vi "findDirectPath.vi"(8 "error in (no error)":errorcluster, 10 "goal platform":i32, 11 "start platform":i32) -> (0 "error out":errorcluster, 1 "vector \nlength":dbl, 2 "vector\nangle":dbl, 3 "path":dbl[](array[numeric]))   [LabVIEW 2017]
panel:
  out "empty?":bool
  out "direct path - first index is row\nof paths through start, \nsecond is location of \ngoal in path":i32[][](array[numeric])
  out "start indices":i32[](array[numeric])
  out "goal indices":i32[](array[numeric])
  out "paths through goal":dbl[][](array[numeric])
  out "paths through start":dbl[][](array[numeric])
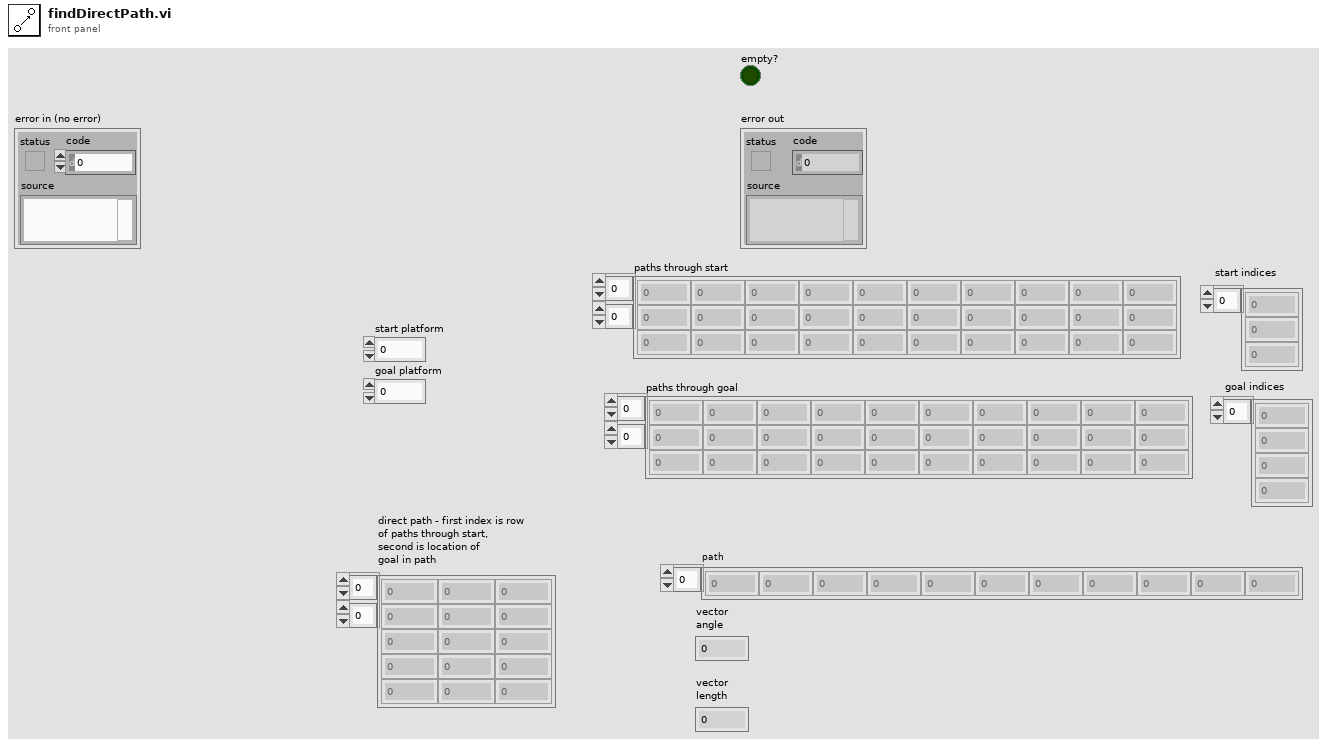
[diagram p1: front panel]
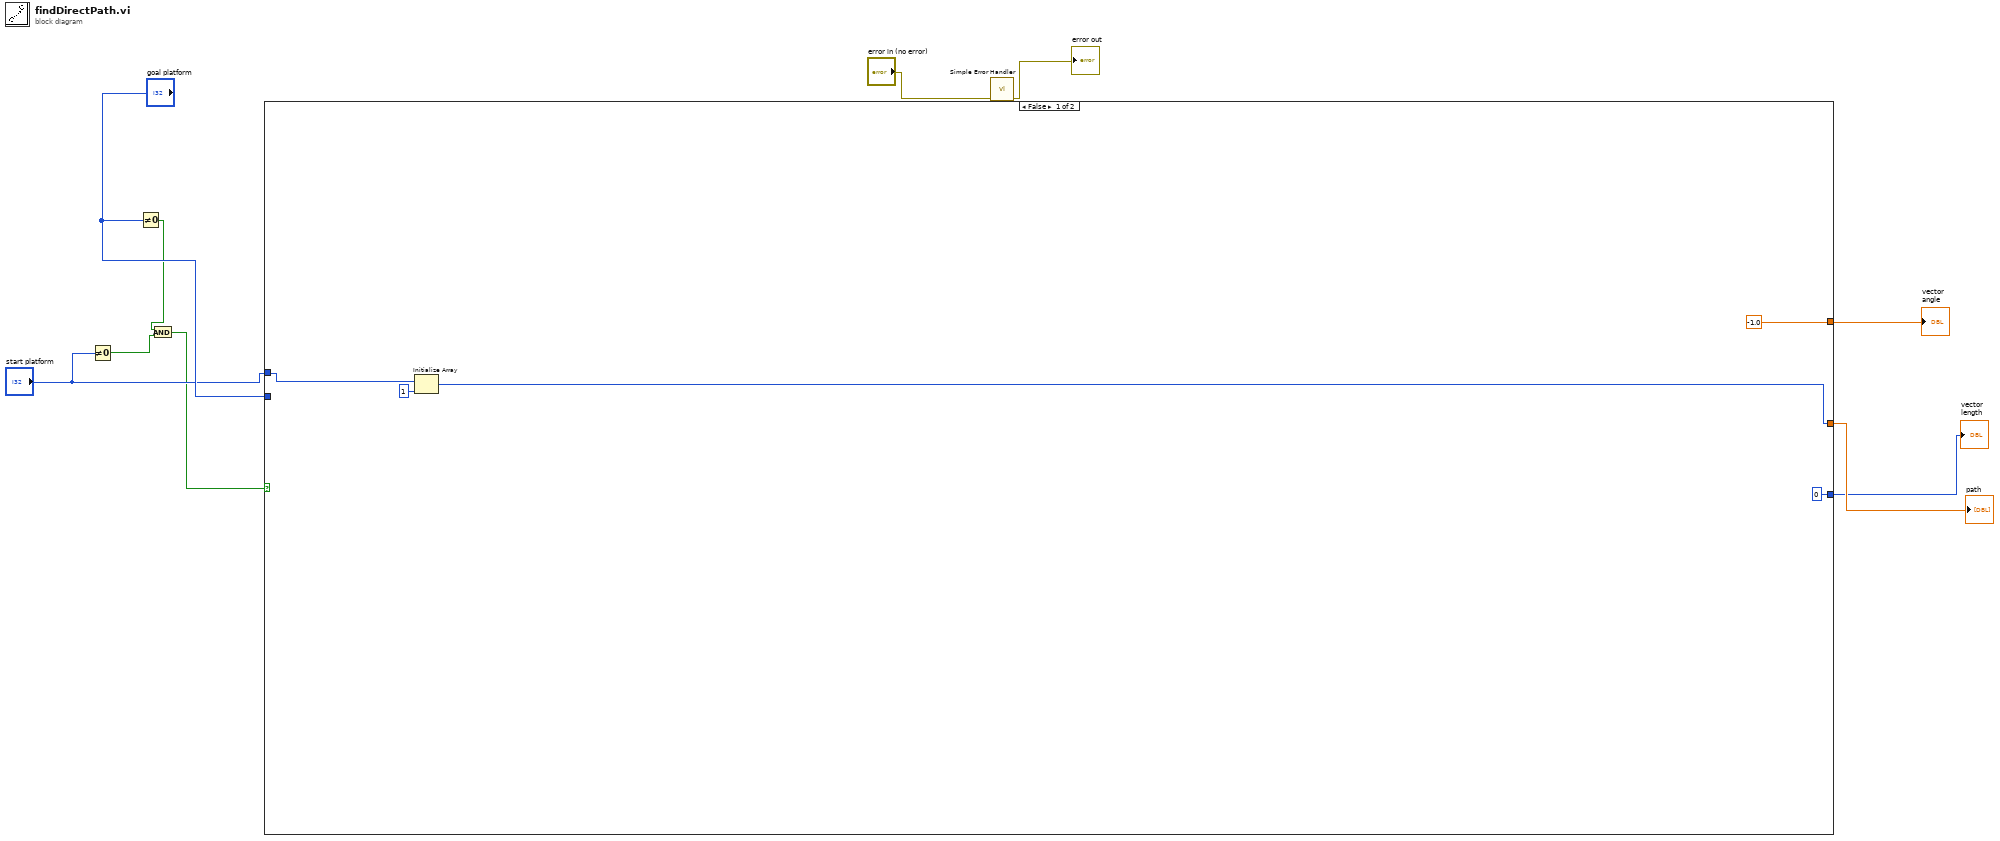
[diagram p0: block diagram]
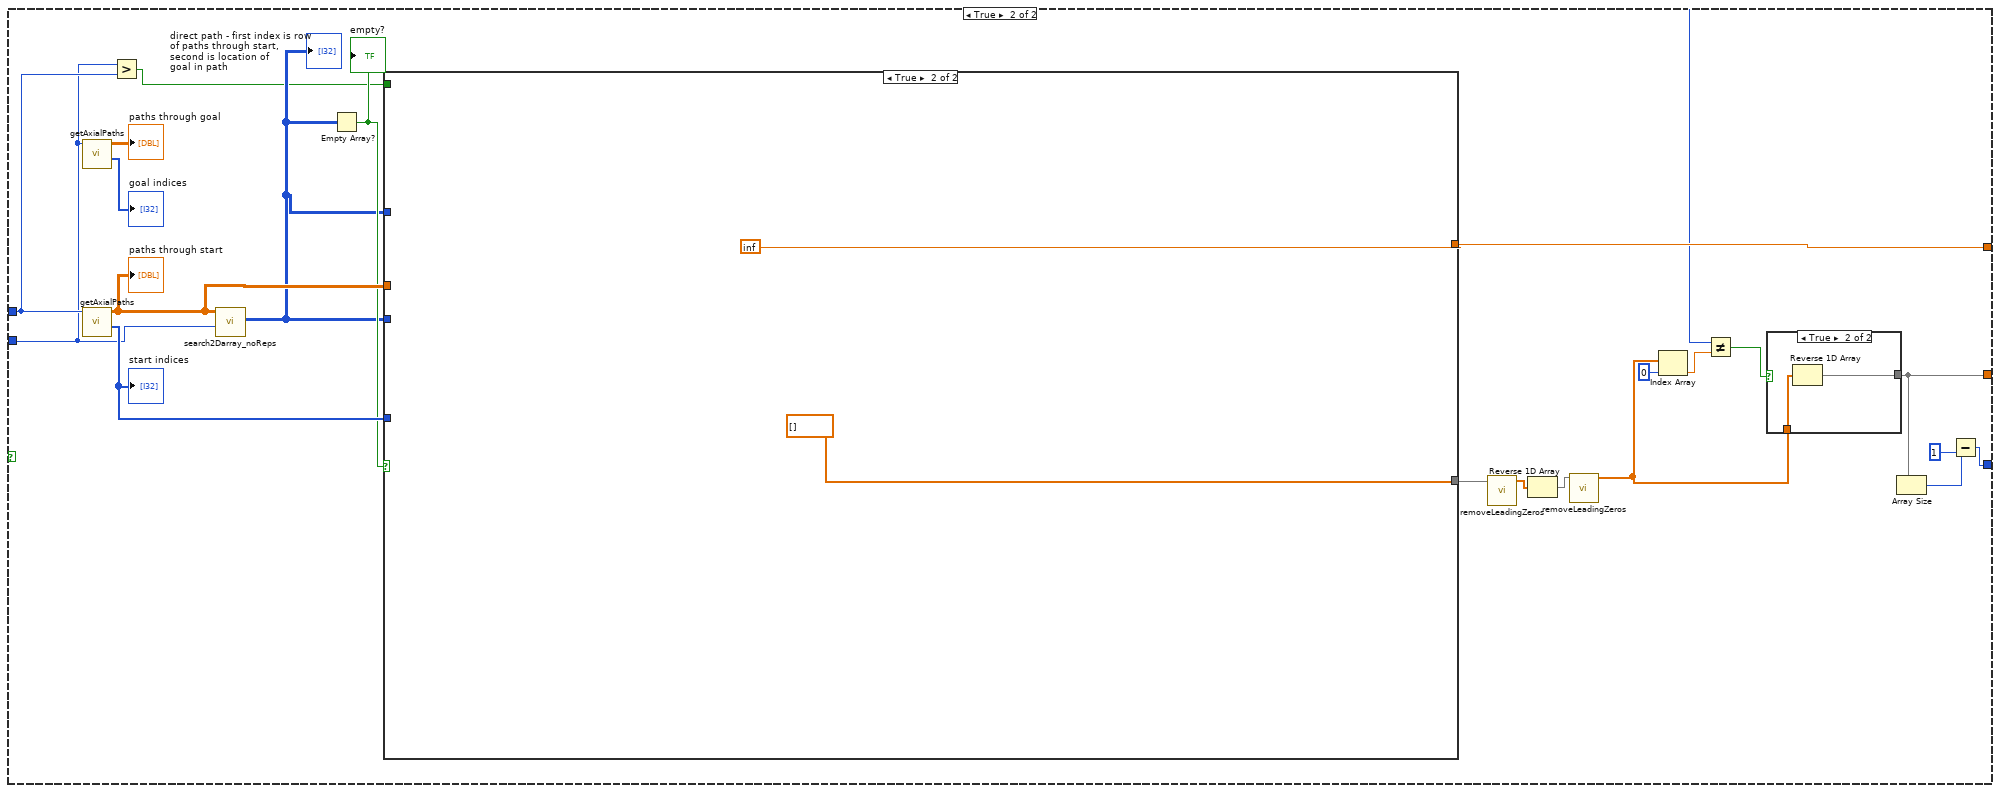
[diagram p2: hidden frame]
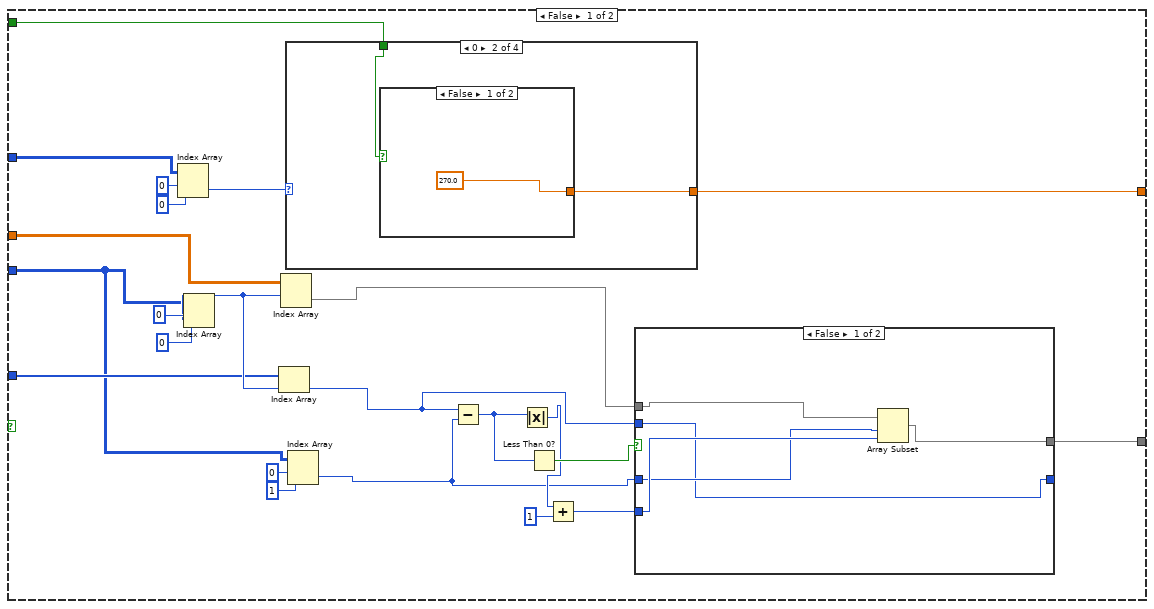
[diagram p4: hidden frame]
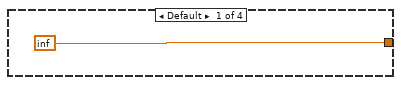
[diagram p5: hidden frame]
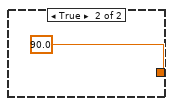
[diagram p6: hidden frame]
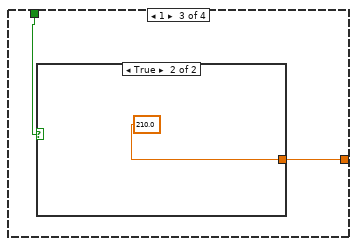
[diagram p7: hidden frame]
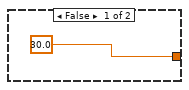
[diagram p8: hidden frame]
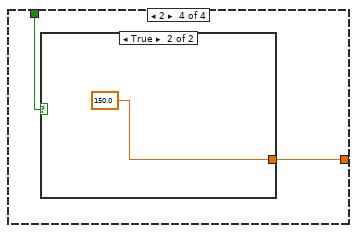
[diagram p9: hidden frame]
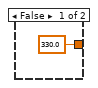
[diagram p10: hidden frame]
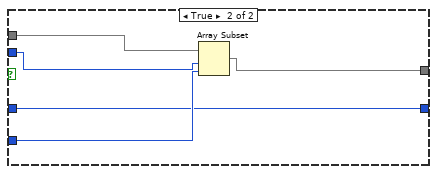
[diagram p11: hidden frame]
diagram:
  n1 = Not Equal To 0?(x="start platform") -> (x != 0?=w2:bool)
  n2 = Not Equal To 0?(x="goal platform") -> (x != 0?=w3:bool)
  n3 = And(x=w3, y=w2) -> (x .and. y?=w1:bool)
  n4 = case shown="False" w1 {
    tunnel: [-1.0 w27] -> w9
    tunnel: "start platform" -> [w13 w26]
    tunnel: [w11 w24] -> w8
    tunnel: "goal platform" -> [_ w23]
    tunnel: [0 w16] -> w5
    frame False {
      n5 = Initialize Array(w13, 1 ("dimension size")) -> (w11:i32[])
    }
    frame True {
      n6 = call "getAxialPaths.vi"("platform"=w23) -> ("platform indices"=→"goal indices":i32[], "paths through start"=→"paths through goal":dbl[][])  [unwired: 9 in]
      n7 = call "getAxialPaths.vi"("platform"=w26) -> ("platform indices"=w33:i32[], "paths through start"=w34:dbl[][])  [unwired: 9 in]
      "paths through start" <- w34
      "start indices" <- w33
      n8 = Greater?(x=w23, y=w26) -> (0:w25:bool)
      n9 = call "search2Darray_noReps.vi"("target"=w23, "Array"=w34) -> ("indices"=w28:i32[][])  [unwired: 9 in]
      "direct path - first index is row\nof paths through start, \nsecond is location of \ngoal in path" <- w28
      n10 = Empty Array?(array=w28) -> (empty?=w32:bool)
      "empty?" <- w32
      n11 = case shown="True" w32 {
        tunnel: w34 -> [w62 _]
        tunnel: w33 -> [w58 _]
        tunnel: w28 -> [w47 _]
        tunnel: [w46 dbl[] []] -> w22
        tunnel: w28 -> [w45 _]
        tunnel: [w41 inf] -> w27
        tunnel: w25 -> [w40 _]
        frame False {
          n12 = Index Array(array=w45, index (row)=0, index (col)=0 ("disabled index (col)")) -> (element=w42:i32)
          n13 = Index Array(array=w47, index (row)=0, index (col)=0 ("disabled index (col)")) -> (element=w59:i32)
          n14 = Index Array(array=w58, index=w59) -> (element=w52:i32)
          n15 = Index Array(array=w62, index (row)=w59) -> (element=w53:dbl[])  [unwired: 1 in]
          n16 = case shown="0" w42 {
            tunnel: [inf w65 w69 w73] -> w41
            tunnel: w40 -> [_ w64 w68 w72]
            frame Default {
            }
            frame 0 {
              n17 = case shown="False" w64 {
                tunnel: [270.0 90.0] -> w65
                frame False {
                }
                frame True {
                }
              }
            }
            frame 1 {
              n18 = case shown="True" w68 {
                tunnel: [30.0 210.0] -> w69
                frame False {
                }
                frame True {
                }
              }
            }
            frame 2 {
              n19 = case shown="True" w72 {
                tunnel: [330.0 150.0] -> w73
                frame False {
                }
                frame True {
                }
              }
            }
          }
          n20 = Index Array(array=w47, index (row)=0, index (col)=1) -> (element=w48:i32)
          n21 = Subtract(x=w52, y=w48) -> (x-y=w55:i32)
          n22 = Absolute Value(x=w55) -> (abs(x)=w51:i32)
          n23 = Less Than 0?(x=w55) -> (x < 0?=w54:bool)
          n24 = Add(x=w51, y=1) -> (x+y=w49:i32)
          n25 = case shown="False" w54 {
            tunnel: w53 -> [w80 w85]
            tunnel: w52 -> [w77 w84]
            tunnel: w49 -> [w79 w83]
            tunnel: [w76 w82] -> w46
            tunnel: w48 -> [w78 w81]
            tunnel: [w77 w81] -> _
            frame False {
              n26 = Array Subset(array=w80, index=w78, length=w79) -> (w76:dbl[])
            }
            frame True {
              n27 = Array Subset(array=w85, index=w84, length=w83) -> (w82:dbl[])
            }
          }
        }
        frame True {
        }
      }
      n28 = call "removeLeadingZeros.vi"("input"=w22) -> ("output"=w21:dbl[])  [unwired: 10 in]
      n29 = Reverse 1D Array(array=w21) -> (reversed array=w20:dbl[])
      n30 = call "removeLeadingZeros.vi"("input"=w20) -> ("output"=w19:dbl[])  [unwired: 10 in]
      n31 = Index Array(array=w19, index=0) -> (element=w30:dbl)
      n32 = Not Equal?(x=w26, y=w30) -> (x != y?=w29:bool)
      n33 = case shown="True" w29 {
        tunnel: w19 -> [w37 w39]
        tunnel: [w37 w38] -> w24
        frame False {
        }
        frame True {
          n34 = Reverse 1D Array(array=w39) -> (reversed array=w38:dbl[])
        }
      }
      n35 = Array Size(array=w24) -> (size(s)=w17:i32)
      n36 = Subtract(x=w17, y=1) -> (x-y=w16:i32)
    }
  }
  "path" <- w8
  "vector\nangle" <- w9
  "vector \nlength" <- w5
  n37 = call <vilib>:"Simple Error Handler.vi"("error in (no error)"="error in (no error)") -> ("error out"=→"error out":errorcluster)  [unwired: 4 in, 4 out]
